vi "End_ControlPowerRelay.vi"(8 "error in":errorcluster, 11 "ControlPowerRelayTask":refnum<k21>="BTS_ControlPower_Relay") -> (0 "error out":errorcluster)   [LabVIEW 2022 SP3]
doc: "This VI will clear the control power relay task"
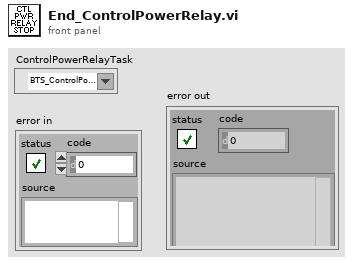
[diagram p1: front panel]
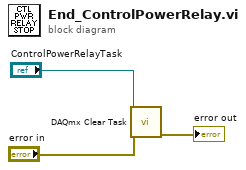
[diagram p0: block diagram]
diagram:
  n1 = call <vilib>:"DAQmx Clear Task.vi"("task in"="ControlPowerRelayTask", "error in"="error in") -> ("error out"=→"error out":errorcluster)  [unwired: 13 in]
